vi "Flush.vi"(6 "returnNodes":bool, 8 "error in (no error)":errorcluster, 11 "LinkedList in":refnum<class "LinkedList.lvclass">) -> (0 "error out":errorcluster, 2 "Nodes":refnum<data-value>[](array[refnum]), 3 "LinkedList out":refnum<class "LinkedList.lvclass">)   [LabVIEW 2009, in "LinkedList.lvclass"]
uses:
  LinkedList.lvclass
  LLNode/LLNode.lvclass
  LinkedList.lvclass/LinkedList.ctl
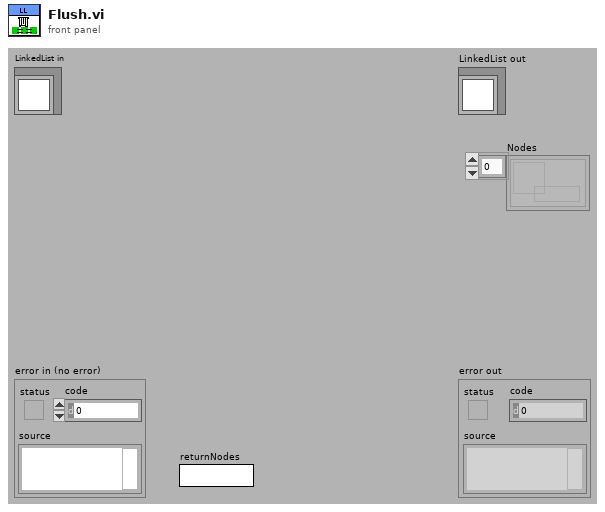
[diagram p1: front panel]
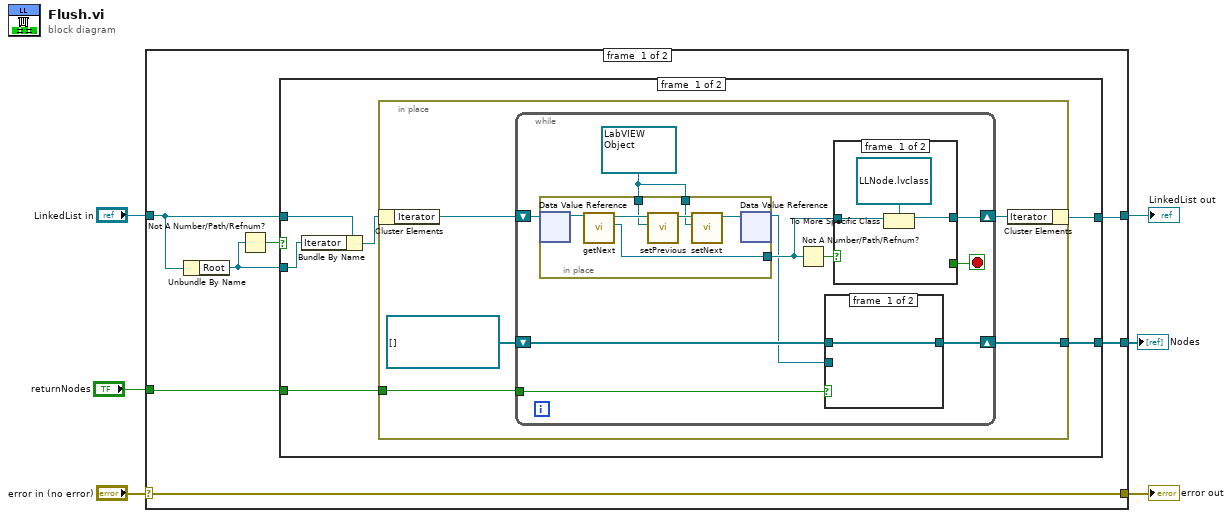
[diagram p0: block diagram]
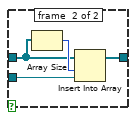
[diagram p2: hidden frame]
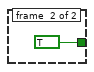
[diagram p3: hidden frame]
diagram:
  n1 = case shown="No Error" "error in (no error)" {
    selector: "error in (no error)" -> [w13 w53]
    tunnel: [w13 w53] -> w5
    tunnel: [w9 w52] -> w3
    tunnel: "LinkedList in" -> [w11 w52]
    tunnel: "returnNodes" -> [w8 _]
    tunnel: [w7 _] -> w1
    frame #0 {
      n2 = Unbundle By Name(w11) -> ("Root"=w10:refnum<data-value>)
      n3 = Not A Number/Path/Refnum?(number/path/refnum=w10) -> (NaN/Path/Refnum?=w12:bool)
      n4 = case shown="False" w12 {
        tunnel: w11 -> [w18 w51]
        tunnel: w10 -> [w19 _]
        tunnel: [w16 w51] -> w9
        tunnel: w8 -> [w15 _]
        tunnel: [w14 _] -> w7
        frame #0 {
          n5 = Bundle By Name(cluster=w18, "Iterator"=w19) -> (w17:refnum<class "LinkedList.lvclass">)
          n6 = in-place {
            in-place-border: w15 -> [w21]
            in-place-border: [w20] -> w14
            n7 = in-place-cluster #1(w17) -> ("Iterator"=w24:refnum<data-value>)
            n8 = while {
              shift-right: [w30] -> w23
              shift-left: w24 -> [w34]
              shift-right: [w26] -> w20
              shift-left: refnum<data-value>[] [] -> [w27]
              tunnel: w21 -> [w28]
              stop <- w32 stop-if-true
              w29 = refnum<data-value> refnum ("previous")
              n9 = in-place {
                in-place-border: [w49] -> w31
                in-place-border: w29 -> [w45]
                in-place-border: w29 -> [w44]
                n10 = in-place-dvr #2(w34) -> (w50:refnum<class "LLNode.lvclass">)  [unwired: 1 out]
                n11 = call "getNext.vi"("LLNode in"=w50) -> ("next"=w49:refnum<data-value>, "LLNode out"=w48:refnum<class "LLNode.lvclass">)  [unwired: 8 in, 1 out]
                n12 = call "setPrevious.vi"("previous"=w45, "LLNode in"=w48) -> ("LLNode out"=w47:refnum<class "LLNode.lvclass">)  [unwired: 8 in, 1 out]
                n13 = call "setNext.vi"("next"=w44, "LLNode in"=w47) -> ("LLNode out"=w46:refnum<class "LLNode.lvclass">)  [unwired: 8 in, 1 out]
                n14 = in-place-dvr #2(w46) -> (w25:refnum<data-value>)  [unwired: 1 out]
              }
              n15 = Not A Number/Path/Refnum?(number/path/refnum=w31) -> (NaN/Path/Refnum?=w33:bool)
              n16 = case shown="True" w28 {
                tunnel: w27 -> [w35 w36]
                tunnel: [w35 w39] -> w26
                tunnel: w25 -> [_ w38]
                frame #0 {
                }
                frame #1 {
                  n17 = Array Size(array=w36) -> (size(s)=w37:i32)
                  n18 = Insert Into Array(array=w36, index=w37, new element=w38) -> (w39:refnum<data-value>[])
                }
              }
              n19 = case shown="True" w33 {
                tunnel: [_ TRUE] -> w32
                tunnel: w31 -> [w42 _]
                tunnel: [w41 _] -> w30
                frame #0 {
                  n20 = To More Specific Class(target class=refnum<data-value> refnum ("Root"), reference=w42) -> (specific class reference=w41:refnum<data-value>)  [unwired: 1 in, 1 out]
                }
                frame #1 {
                }
              }
            }
            n21 = in-place-cluster #1("Iterator"=w23) -> (w16:refnum<class "LinkedList.lvclass">)
          }
        }
        frame #1 {
        }
      }
    }
    frame #1 {
    }
  }
  "error out" <- w5
  "LinkedList out" <- w3
  "Nodes" <- w1
